vi "Schedule Guardian Recheck.vi"(8 "error in (no error)":errorcluster, 10 "Guardian ID":string, 11 "Guardian in":refnum<class "Guardian.lvclass">) -> (0 "error out":errorcluster, 3 "Guardian out":refnum<class "Guardian.lvclass">)   [LabVIEW 2026, in "TALOS.lvlib" / "Guardian.lvlib" / "Guardian.lvclass"]
uses:
  Guardian.lvclass
  C:/LabVIEW Code/TALOS/builds/Actor Framework PPL/Actor Framework.lvlibp/1abvi3w/vi.lib/ActorFramework/Actor/Actor.lvclass
  builds/Actor Framework PPL/Actor Framework.lvlibp/1abvi3w/vi.lib/ActorFramework/Message Enqueuer/Message Priority.ctl
  Guardian Messages/Guardian Died Recheck Msg/Guardian Died Recheck Msg.lvclass
  C:/LabVIEW Code/TALOS/builds/Actor Framework PPL/Actor Framework.lvlibp/1abvi3w/vi.lib/ActorFramework/Message/Message.lvclass
  Guardian Messages/Guardian Died Recheck Msg/Guardian Died Recheck Msg.lvclass/Guardian Died Recheck Msg.ctl
  Ancestor/Ancestor/Ancestor.lvclass/Ancestor.ctl
  Support VIs/Generate Error.vi
  FGV/Error Memory/Get Error Description.vi
  Support VIs/Get PC name.vi
  Ancestor/Ancestor/Read ID.vi
  Support VIs/Get Class Name.vi
  <vilib>/Utility/error.llb/Clear Errors.vi
  FGV/Error Memory/Error Memory Core.vi
  <vilib>/AdvancedString/Delimited String to 1D String Array.vi
  <vilib>/AdvancedString/Delimited String to 1D String Array (string).vi
  Support VIs/Circus Root Path.vi
  FGV/Error Memory/Error Crt Lvl checker.vi
  FGV/Error Memory/Error Memory Core.vi/40c8088d-b597-4017-91af-faa98e00292e.vi
  FGV/Error Memory/Error Memory Core.vi/d4a3ab98-063c-4e44-b43d-fbdcfe6c2be2.vi
  Support VIs/Global Memory.vi
  <vilib>/Utility/LVClass/Get LV Class Name.vi
  Support VIs/Is in Packed Library.vi
  Support VIs/TALOS Root path.vi
  Support VIs/Read CSV worksheet.vi
  Support VIs/Global Constants.vi
  <vilib>/Utility/error.llb/General Error Handler.vi
  <vilib>/Utility/config.llb/Open Config Data.vi
  <vilib>/Utility/config.llb/Get Section Names.vi
  <vilib>/Utility/config.llb/Get Key Names.vi
  <vilib>/Utility/config.llb/Read Key.vi
  <vilib>/Utility/config.llb/Read Key (String).vi
  <vilib>/Utility/config.llb/Close Config Data.vi
  Support VIs/Error Log.vi
  Ancestor/Ancestor/Ancestor.lvclass
  <vilib>/Comparison/Equal/Equal Functor/Equal Functor.lvclass
  builds/Actor Framework PPL/Actor Framework.lvlibp/1abvi3w/vi.lib/ActorFramework/Actor/Actor.lvclass
  builds/Actor Framework PPL/Actor Framework.lvlibp
  builds/Actor Framework PPL/Actor Framework.lvlibp/1abvi3w/vi.lib/ActorFramework/Message Enqueuer/Message Enqueuer.lvclass
  TALOS.lvlib
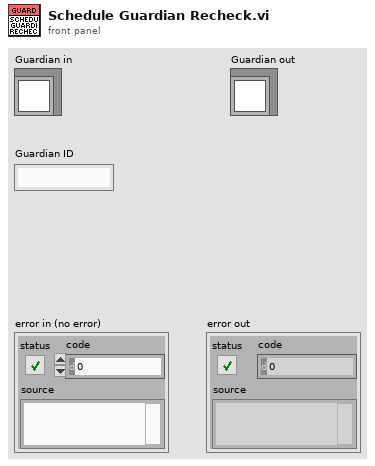
[diagram p1: front panel]
types:
  T1 = typedef "Actor Framework.lvlibp/Message Enqueuer.lvclass/Message Priority.ctl" = enum16{"Low", "Normal", "High"}
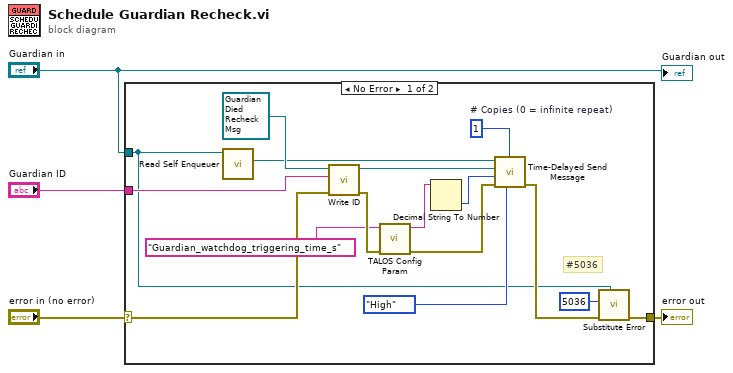
[diagram p0: block diagram]
diagram:
  n1 = case shown="No Error" "error in (no error)" {
    selector: "error in (no error)" -> [w18 w21]
    tunnel: "Guardian in" -> [w6 _]
    tunnel: [w7 w21] -> w4
    tunnel: "Guardian ID" -> [w19 _]
    frame No Error {
      w15 = u32 1  # # Copies (0 = infinite repeat)
      # "#5036"
      n2 = call "Read Self Enqueuer.vi"("Actor"=w6) -> ("Self Enqueuer"=w16:refnum<class "Message Enqueuer.lvclass">)  [unwired: 10 in]
      n3 = call "Write ID.vi"("error in (no error)"=w18, "ID"=w19, "Guardian Died Recheck Msg in"=refnum<class "Guardian Died Recheck Msg.lvclass"> refnum ("Guardian.lvlib:Guardian Died Recheck Msg.lvclass")) -> ("error out"=w12:errorcluster, "Guardian Died Recheck Msg out"=w17:refnum<class "Guardian Died Recheck Msg.lvclass">)  [unwired: 7 in]
      n4 = call "TALOS Config Param.vi"("error in (no error)"=w12, "Parameter Name"="Guardian_watchdog_triggering_time_s") -> ("error out"=w11:errorcluster, "Output"=w10:string)  [unwired: 8 in]
      n5 = Decimal String To Number(string=w10) -> (number=w13:i32)  [unwired: 2 in, 1 out]
      n6 = call "Time-Delayed Send Message.vi"("Message Priority (Normal)"=Message_Priority."High", "# Copies (0 = infinite repeat)"=w15, "error in (no error)"=w11, "Milliseconds To Wait"=w13, "Message"=w17, "Message Enqueuer"=w16) -> ("error out"=w8:errorcluster)  [unwired: 4 in, 1 out]
      n7 = call "Substitute Error.vi"("LabVIEW Object"=w6, "error in (no error)"=w8, "Error Code"=5036) -> ("error out"=w7:errorcluster)  [unwired: 8 in]
    }
    frame Error {
    }
  }
  "error out" <- w4
  "Guardian out" <- "Guardian in"
